vi "PruneSelection.vi"(6 "maxFileCount":i32, 8 "error in (no error)":errorcluster, 11 "ExistingFiles":path[](array[path])) -> (0 "error out":errorcluster, 3 "FilesToDelete":path[](array[path]))   [LabVIEW 2026, in "Lumberjack.lvlib"]
doc: "Pure retention selection. Group the existing files by base name, then within each group keep the newest MaxFileCount (ordered by embedded ISO 8601 timestamp) and return the rest for deletion. Prunes only when MaxFileCount is positive; any non-positive value (including the -1 unbounded sentinel) keeps all and returns none (SRS-LMBR-034). Selects only; deletion happens in FileAppender:Prune. Deterministic; no I/O.\n\nPer-base-name: keep newest MaxFileCount (>0); non-positive keeps all."
uses:
  Lumberjack.lvlib
  <vilib>/regexp/Match Regular Expression.xnode
panel:
  out "Numeric":i32
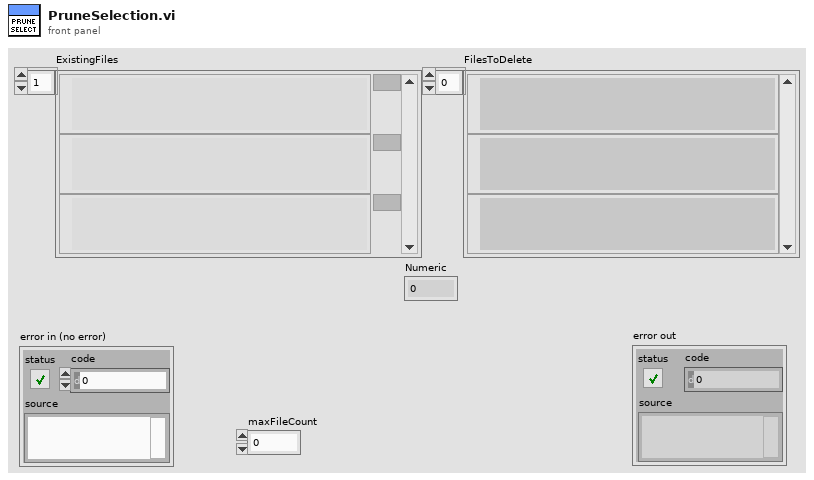
[diagram p1: front panel]
types:
  T1 = cluster{"BaseName":string, "TimeKey":string, "Path":path}
  T2 = cluster{"BaseName":string, "TimeKey":string, "Path":path}[]
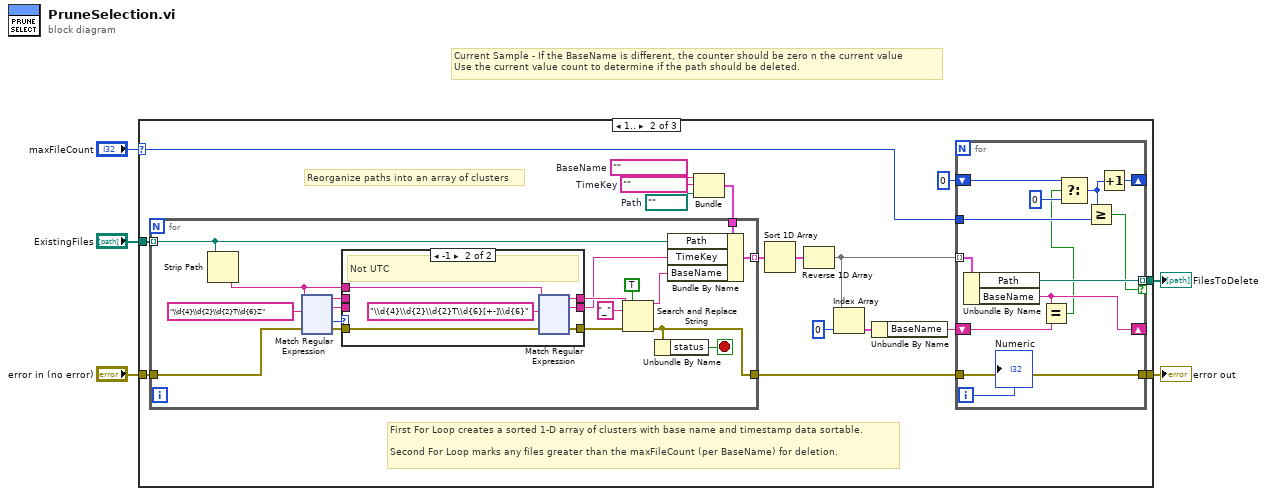
[diagram p0: block diagram]
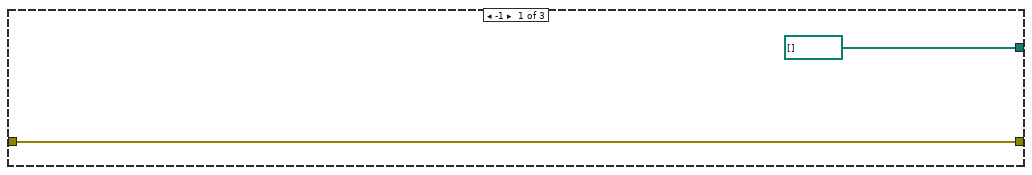
[diagram p2: hidden frame]
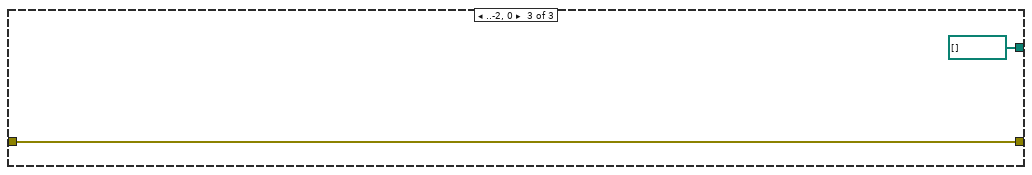
[diagram p4: hidden frame]
diagram:
  # "Current Sample - If the BaseName is different, the counter should be zero n the current value\nUse the current value count to determine if the path should be deleted."
  n1 = case shown="1.." "maxFileCount" {
    selector: "maxFileCount" -> [_ w10 _]
    tunnel: "ExistingFiles" -> [_ w24 _]
    tunnel: "error in (no error)" -> [w6 w19 w300]
    tunnel: [path[] [] ("ExistingFiles") w9 path[] [] ("ExistingFiles")] -> w1
    tunnel: [w6 w8 w300] -> w2
    frame -1 {
    }
    frame 1.. {
      w22 = ""  # TimeKey
      w21 = path ""  # Path
      w23 = ""  # BaseName
      # "First For Loop creates a sorted 1-D array of clusters with base name and timestamp data sortable.\n\nSecond For Loop marks any files greater than the maxFileCount (per BaseName) for deletion."
      # "Reorganize paths into an array of clusters"
      n2 = Bundle("BaseName"=w23, "TimeKey"=w22, "Path"=w21) -> (w20:T1)  [unwired: 1 in]
      n3 = for {
        tunnel: w24 -> [w54] mode=indexing
        tunnel: w20 -> [w55]
        tunnel: w19 -> [w51]
        tunnel: [w39] -> w16
        tunnel: [w45] -> w17 mode=indexing
        stop <- w52 stop-if-true
        n4 = Strip Path(path=w54) -> (name=w46:string)  [unwired: 1 out]
        n5 = xnode "Match Regular Expression"("input string"=w46, "regular expression"="\\d{4}\\d{2}\\d{2}T\\d{6}Z", "error in"=w51) -> ("before match"=w47:string, "whole match"=w48:string, "offset past match"=w50:i32, "error out"=w49:errorcluster)  [unwired: 3 in, 1 out]
        n6 = case shown="-1" w50 {
          tunnel: w49 -> [w57 w64]
          tunnel: w48 -> [w58 _]
          tunnel: [w58 w60] -> w38
          tunnel: w47 -> [w56 _]
          tunnel: [w57 w61] -> w42
          tunnel: w46 -> [_ w63]
          tunnel: [w56 w59] -> w44
          frame 0, Default {
            # "UTC"
          }
          frame -1 {
            # "Not UTC"
            n7 = xnode "Match Regular Expression"("input string"=w63, "regular expression"="\\d{4}\\d{2}\\d{2}T\\d{6}[+-]\\d{6}", "error in"=w64) -> ("before match"=w59:string, "whole match"=w60:string, "error out"=w61:errorcluster)  [unwired: 3 in, 2 out]
          }
        }
        n8 = Search and Replace String(replace all?=TRUE ("replace all? (F)"), input string=w44, search string="_", error in=w42) -> (result string=w40:string, error out=w39:errorcluster)  [unwired: 4 in, 2 out]
        n9 = Unbundle By Name(w39) -> ("status"=w52:bool)
        n10 = Bundle By Name(cluster=w55, "Path"=w54, "TimeKey"=w38, "BaseName"=w40) -> (w45:T1)
      }
      n11 = Sort 1D Array(array=w17) -> (sorted array=w18:T2)
      n12 = Reverse 1D Array(array=w18) -> (reversed array=w15:T2)
      n13 = Index Array(array=w15, index=0) -> (element=w12:T1)
      n14 = Unbundle By Name(w12) -> ("BaseName"=w11:string)
      n15 = for {
        tunnel: w15 -> [w37] mode=indexing
        tunnel: w16 -> [w32]
        shift-right: [w31] -> _
        shift-left: w11 -> [w36]
        shift-right: [w26] -> _
        shift-left: 0 ("index") -> [w25]
        tunnel: w10 -> [w34]
        tunnel: [w33] -> w9 mode=indexing if=w30
        tunnel: [w32] -> w8
        i -> [w28]
        n16 = Unbundle By Name(w37) -> ("Path"=w33:path, "BaseName"=w31:string)
        n17 = Equal?(x=w31, y=w36) -> (x = y?=w29:bool)
        n18 = Select(t=w25, s=w29, f=0) -> (s? t:f=w27:i32)
        n19 = Greater Or Equal?(x=w27, y=w34) -> (x >= y?=w30:bool)
        n20 = Increment(x=w27) -> (x+1=w26:i32)
        "Numeric" <- w28
      }
    }
    frame ..-2, 0 {
    }
  }
  "FilesToDelete" <- w1
  "error out" <- w2
